vi "Read Unsigned Integer Configuration.vi"(7 "Type":T1, 8 "error in (no error)":errorcluster, 9 "Default If Not Found":u64, 10 "Name":string, 11 "database-configuration in":refnum<class "configuration-database.lvclass">) -> (0 "error out":errorcluster, 1 "Not Found?":bool, 2 "Value":u64, 3 "database-configuration out":refnum<class "configuration-database.lvclass">)   [LabVIEW 2020, in "configuration-database.lvlib" / "configuration-database.lvclass"]
uses:
  configuration-database.lvclass
  <vilib>/Utility/Data Type/Type Definitions/Data Type.ctl
  configuration-database.lvclass/configuration-database.ctl
  8683f4a9-b319-4472-8d6f-9168a35df6e1.vi
  8683f4a9-b319-4472-8d6f-9168a35df6e1.vi/82966b15-8689-4d97-9a0e-bd5327f0291f.vi
  <vilib>/Utility/error.llb/Error Cluster From Error Code.vi
  IConfigDBQueries/IConfigurationDatabaseQueries.lvclass
  <vilib>/ErrorRing/Error Ring.xnode
  externals/database-interface/IDatabase/IDatabase/IDatabase.lvclass
  <vilib>/Utility/Data Type/NI_Data Type.lvlib
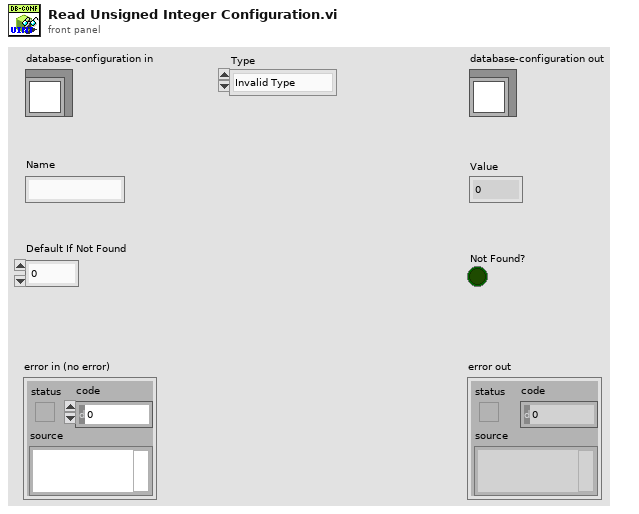
[diagram p1: front panel]
types:
  T1 = typedef "NI_Data Type.lvlib/Data Type.ctl" = enum8{"Invalid Type", "Void", "I8", "I16", "I32", "I64", "U8", "U16", "U32", "U64", "Single Float", "Double Float", "Extended Float", "Single Complex", "Double Complex", "Extended Complex", "Enum U8", "Enum U16", "Enum U32", "Enum U64", "Single Float With Unit", "Double Float With Unit", "Extended Float With Unit", "Single Complex with Unit", "Double Complex with Unit", "Extended Complex with Unit", "Boolean", "String", "Path", "Picture", "Tag", "Array", "Cluster", "Variant", "LV Variant", "Waveform", "Timestamp", "Digital Waveform", "Digital Data", "ExpressData", "Refnum", "External Data", "VI", "Poly VI", "LabVIEW Class Instance", "Fixed Point", "Set Collection", "Map Collection"}
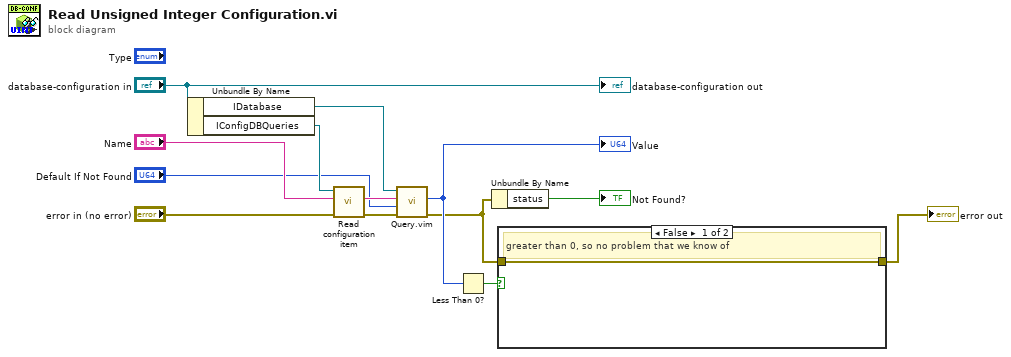
[diagram p0: block diagram]
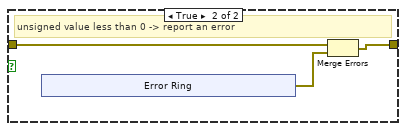
[diagram p2: hidden frame]
diagram:
  n1 = Unbundle By Name("database-configuration in") -> ("IDatabase"=w12:refnum<class "IDatabase.lvclass">, "IConfigDBQueries"=w13:refnum<class "IConfigurationDatabaseQueries.lvclass">)
  n2 = call-dynamic "Read configuration item.vi"("error in (no error)"="error in (no error)", "configuration item"="Name", "IConfigDBQueries in"=w13) -> ("error out"=w11:errorcluster, "result"=w10:string)  [unwired: 7 in]
  n3 = call "Query.vim"("error in (no error)"=w11, "Type and Default"="Default If Not Found", "Query string"=w10, "IDatabase in"=w12) -> ("error out"=w1:errorcluster, "Result"=w2:u64)  [unwired: 5 in, 1 out]
  "Value" <- w2
  n4 = Less Than 0?(x=w2) -> (x < 0?=w5:bool)
  n5 = Unbundle By Name(w1) -> ("status"=→"Not Found?":bool)
  n6 = case shown="False" w5 {
    tunnel: w1 -> [w14 w17]
    tunnel: [w14 w16] -> w4
    frame False {
      # "greater than 0, so no problem that we know of"
    }
    frame True {
      # "unsigned value less than 0 -> report an error"
      n7 = xnode "Error Ring"() -> ("error out"=w15:errorcluster)
      n8 = Merge Errors(w17, w15) -> (w16:errorcluster)
    }
  }
  "error out" <- w4
  "database-configuration out" <- "database-configuration in"
